vi "PFMate-Dual.vi"() -> ()   [LabVIEW 2009]
uses:
  <vilib>/NXT/Subs/LVHSConnector.ctl
  <vilib>/NXT/Block Support/NXT_InputPort.ctl
  mindsensors.com LVEE Toolkit/Dual/PFMate-DM.vi
panel:
  in  "Inputs":T1={"Dir A"=TRUE, "MA"=0, "MB"=0, "Operation"=0, "Pwr A"=5, "Pwr B"=5, "Dir B"=TRUE, "Channel"=1, "PFMate address 2"=72} {"PFMate address 2" format="%x"; "Pwr B" min=1 max=7 step=1 scale=1.0..7.0; "Pwr A" min=1 max=7 step=1 scale=1.0..7.0; "MB" items=["Run", "Float", "Brake"]; "MA" items=["Run", "Float", "Brake"]}
  in  "Input Port":T2 items=["Port 1", "Port 2", "Port 3", "Port 4"]
  out "NXT dup":T3={"error"={"status"=FALSE, "code"=0, "source"=""}, "address"="", "NXT #"=-1, "Show Error"=TRUE}
  in  "NXT":T3={"error"={"status"=FALSE, "code"=0, "source"=""}, "address"="", "NXT #"=-1, "Show Error"=TRUE}
  in  "stop":bool
  # "mindsensors.com\nCopyright (c) 2009 by mindsensors.com\nEmail: info (<at>) mindsensors (<dot>) com\n\nThis program is free software. You can redistribute it and/or modify\nit under the terms of the GNU General Public License as published by\nthe Free Software Foundation; version 3 of the License.\nRead the license at: http://www.gnu.org/licenses/gpl.txt"
  # "Motor A"
  # "Motor B"
  # "Mode"
  # "Direction"
  # "Power"
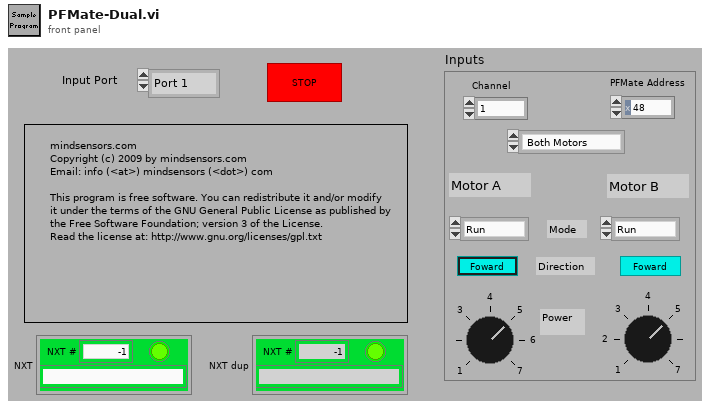
[diagram p1: front panel]
types:
  T1 = cluster{"Dir A":bool, "MA":u8, "MB":u8, "Operation":u8, "Pwr A":u8, "Pwr B":u8, "Dir B":bool, "Channel":u8, "PFMate address 2":u8}
  T2 = typedef "NXT_InputPort.ctl" = u8
  T3 = typedef "LVHSConnector.ctl" = cluster{"error":errorcluster, "address":string, "NXT #":i32, "Show Error":bool}
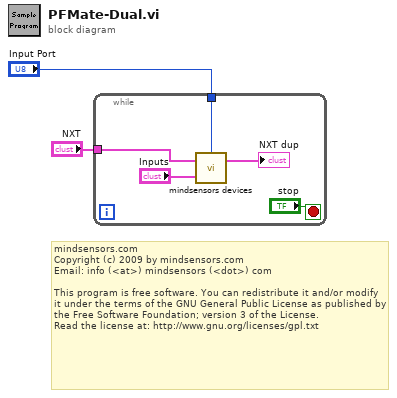
[diagram p0: block diagram]
diagram:
  # "mindsensors.com\nCopyright (c) 2009 by mindsensors.com\nEmail: info (<at>) mindsensors (<dot>) com\n\nThis program is free software. You can redistribute it and/or modify\nit under the terms of the GNU General Public License as published by\nthe Free Software Foundation; version 3 of the License.\nRead the license at: http://www.gnu.org/licenses/gpl.txt"
  n1 = while {
    tunnel: "NXT" -> [w6]
    tunnel: "Input Port" -> [w4]
    stop <- "stop" stop-if-true
    n2 = call-poly "mindsensors devices.vi"("Inputs"="Inputs", "NXT"=w6, "Input Port"=w4) -> ("NXT dup"=→"NXT dup":T3)  [unwired: 1 in]
  }
